vi "F05 Config.vi"(6 "Frequency(Hz)":dbl=1000.0, 7 "Offset(V)":dbl, 8 "error in (no error)":errorcluster, 9 "Amplitude(Vp-p)":dbl=5.0, 10 "Waveform Mode":T1(ring), 11 "MyIndex":u8) -> (0 "error out":errorcluster, 3 "Pass/Fail":bool)   [LabVIEW 2015]
uses:
  <vilib>/Instr/_visa.llb/VISA Configure Serial Port (Instr).vi
panel:
  out "VISA":refnum<visa-resource-name> caption="VISA资源名称输出"
  out "resulting string":string
  # "Config the F05"
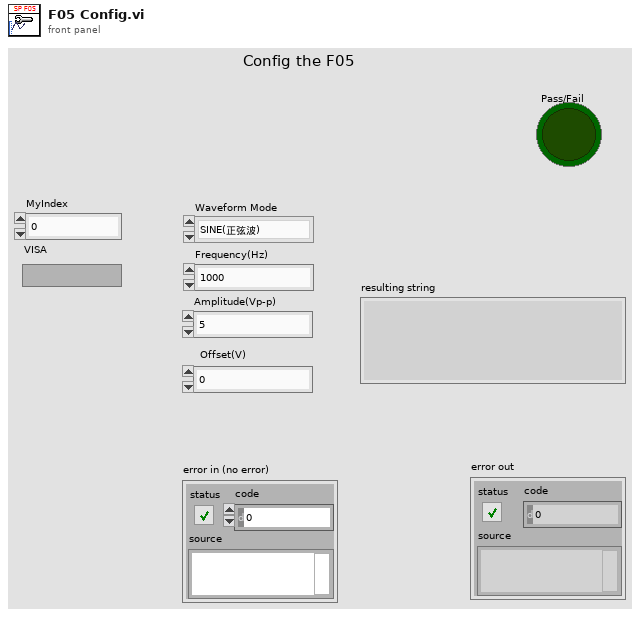
[diagram p1: front panel]
types:
  T1 = enum16{"SINE(正弦波)", "SQUARE(方波)", "TRIANG(三角波)", "UP_RAMP(升锯齿)", "DOWN_RAMP(降锯齿)", "NOISE(噪声)"}
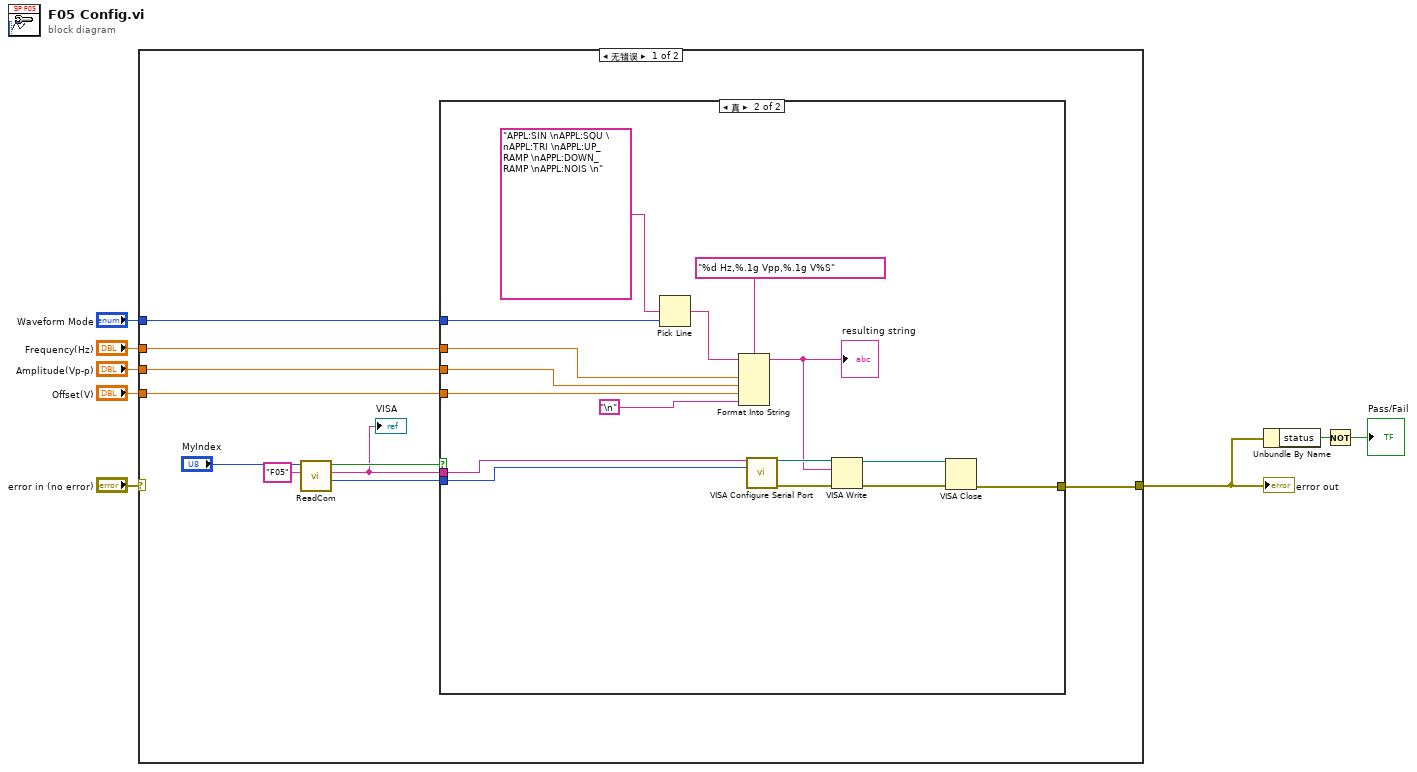
[diagram p0: block diagram]
diagram:
  n1 = case shown="无错误" "error in (no error)" {
    selector: "error in (no error)" -> [_ w35]
    tunnel: [w12 w35] -> w1
    tunnel: "Waveform Mode" -> [w18 _]
    tunnel: "Frequency(Hz)" -> [w17 _]
    tunnel: "Amplitude(Vp-p)" -> [w16 _]
    tunnel: "Offset(V)" -> [w15 _]
    frame No Error {
      n2 = call "ReadCom.vi"("仪器名称"="F05", "MyIndex"="MyIndex") -> ("Baudrate"=w9:i32, "COM"=w10:string, "OK?"=w11:bool)  [unwired: 7 in]
      "VISA" <- w10
      n3 = case shown="真" w11 {
        tunnel: w18 -> [_ w34]
        tunnel: w17 -> [_ w30]
        tunnel: w16 -> [_ w29]
        tunnel: w15 -> [_ w28]
        tunnel: [_ w21] -> w12
        tunnel: w10 -> [_ w20]
        tunnel: w9 -> [_ w19]
        frame False {
        }
        frame True {
          n4 = Pick Line(multi-line string="APPL:SIN \nAPPL:SQU \nAPPL:TRI \nAPPL:UP_RAMP \nAPPL:DOWN_RAMP \nAPPL:NOIS \n", line index=w34) -> (output string=w32:string)  [unwired: 1 in]
          n5 = Format Into String(format string="%d Hz,%.1g Vpp,%.1g V%S", initial string=w32, w30, w29, w28, "\n") -> (resulting string=w24:string)  [unwired: 1 in, 1 out]
          "resulting string" <- w24
          n6 = call-poly "VISA Configure Serial Port"("VISA resource name"=w20, "baud rate (9600)"=w19) -> ("VISA resource name out"=w26:refnum<visa-resource-name>, "error out"=w27:errorcluster)  [unwired: 12 in]
          n7 = VISA Write(VISA resource name=w26, write buffer=w24, error in (no error)=w27) -> (VISA resource name out=w23:refnum<visa-resource-name>, error out=w22:errorcluster)  [unwired: 1 out]
          n8 = VISA Close(VISA resource name=w23, error in (no error)=w22) -> (error out=w21:errorcluster)
        }
      }
    }
    frame Error {
    }
  }
  "error out" <- w1
  n9 = Unbundle By Name(w1) -> ("status"=w3:bool)
  n10 = Not(x=w3) -> (.not. x?=→"Pass/Fail":bool)
